vi "ImageSizeConvert.vi"(1 "Image Size":T1) -> (0 "intImgSizes":cluster{i32, i32})   [LabVIEW 2013]
uses:
  <vilib>/Rock Robotics/WPI/Camera/WPI_CameraImageSize.ctl
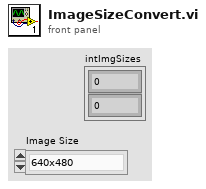
[diagram p1: front panel]
types:
  T1 = typedef "WPI_CameraImageSize.ctl" = enum16{"640x480", "320x240", "160x120"}
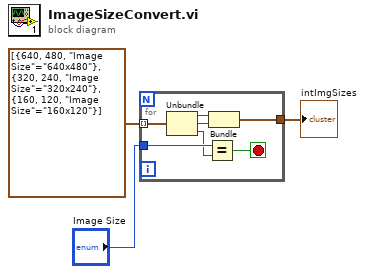
[diagram p0: block diagram]
diagram:
  n1 = for {
    tunnel: "Image Size" -> [w9]
    tunnel: cluster{i32, i32, "Image Size":T1}[] [{640, 480, "Image Size"=enum."640x480"}, {320, 240, "Image Size"=enum."320x240"}, {160, 120, "Image Size"=enum."160x120"}] -> [w10] mode=indexing
    tunnel: [w6] -> w1
    stop <- w7 stop-if-true
    n2 = Unbundle(w10) -> (w4:i32, w5:i32, "Image Size"=w8:T1)
    n3 = Equal?(x=w9, y=w8) -> (x = y?=w7:bool)
    n4 = Bundle(w4, w5) -> (w6:cluster{i32, i32})  [unwired: 1 in]
  }
  "intImgSizes" <- w1
